vi "ElevatorManualControl.vi"(9 "Elevator State":string) -> (0 "Manual Contribution":dbl)   [LabVIEW 2018]
uses:
  Inputs_DriverStation.vi
  RobotStates.vi
  SensorReadings.vi
panel:
  in  "Maximum Climb Height (in)":dbl=150.0
  in  "Bump Down Climb":dbl=0.5
  in  "Bump Up Climb":dbl=0.1
  in  "Bump Up":dbl=0.9
  in  "Bump Down":dbl=0.3
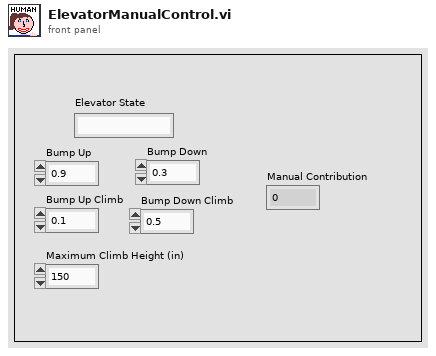
[diagram p1: front panel]
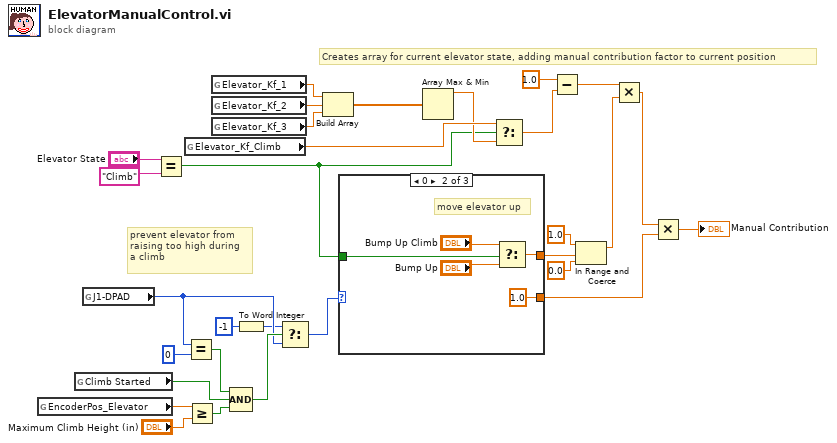
[diagram p0: block diagram]
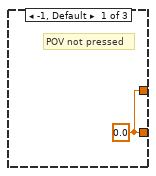
[diagram p2: hidden frame]
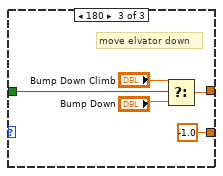
[diagram p3: hidden frame]
diagram:
  # "prevent elevator from\nraising too high during\na climb"
  # "Creates array for current elevator state, adding manual contribution factor to current position"
  n1 = global read "SensorReadings.vi" "EncoderPos_Elevator"() -> (w11:dbl)
  n2 = global read "RobotStates.vi" "Climb Started"() -> (w9:bool)
  n3 = global read "Inputs_DriverStation.vi" "J1-DPAD"() -> (w4:i16)
  n4 = Equal?(x="Elevator State", y="Climb") -> (x = y?=w12:bool)
  n5 = global read "Inputs_DriverStation.vi" "Elevator_Kf_Climb"() -> (w15:dbl)
  n6 = Equal?(x=w4, y=i16 0) -> (x = y?=w8:bool)
  n7 = Greater Or Equal?(x=w11, y="Maximum Climb Height (in)") -> (x >= y?=w10:bool)
  n8 = global read "Inputs_DriverStation.vi" "Elevator_Kf_1"() -> (w21:dbl)
  n9 = global read "Inputs_DriverStation.vi" "Elevator_Kf_2"() -> (w20:dbl)
  n10 = global read "Inputs_DriverStation.vi" "Elevator_Kf_3"() -> (w19:dbl)
  n11 = Compound Arithmetic op=AND(w8, w9, w10) -> (w6:bool)
  n12 = To Word Integer(number=-1) -> (16bit integer=w3:i16)
  n13 = Select(t=w3, s=w6, f=w4) -> (s? t:f=w2:i16)
  n14 = Build Array(w21, w20, w19) -> (w18:dbl[])
  n15 = case shown="0" w2 {
    tunnel: [w31 1.0 -1.0] -> w30
    tunnel: [w31 w35 w40] -> w22
    tunnel: w12 -> [_ w34 w39]
    frame -1, Default {
      w31 = 0.0
      # "POV not pressed"
    }
    frame 0 {
      # "move elevator up"
      n16 = Select(t="Bump Up Climb", s=w34, f="Bump Up") -> (s? t:f=w35:dbl)
    }
    frame 180 {
      # "move elvator down"
      n17 = Select(t="Bump Down Climb", s=w39, f="Bump Down") -> (s? t:f=w40:dbl)
    }
  }
  n18 = Array Max & Min(array=w18) -> (max value=w14:dbl)  [unwired: 3 out]
  n19 = Select(t=w15, s=w12, f=w14) -> (s? t:f=w13:dbl)
  n20 = Subtract(x=1.0, y=w13) -> (x-y=w28:dbl)
  n21 = In Range and Coerce(upper limit=1.0, x=w22, lower limit=0.0) -> (coerced(x)=w23:dbl)  [unwired: 1 out]
  n22 = Multiply(x=w28, y=w23) -> (x*y=w27:dbl)
  n23 = Multiply(x=w27, y=w30) -> (x*y=→"Manual Contribution":dbl)
